vi "XLP80_GUI_PandID.vi"(8 "err in":errorcluster) -> (0 "err out":errorcluster)   [LabVIEW 2021]
uses:
  XLP80_ProjectLibs/XLP80_GUI_V001.llb/XLP80_GUI_TDefClusterPandID_Gen2_FM2.ctl
  XLP80_ProjectLibs/XLP80_GUI_V001.llb/XLP80_GUI_TDefClusterPandID_Gen2_FM1.ctl
  XLP80_ProjectLibs/XLP80_Globals/Globals_Settings_XLP80.vi
  XLP80_General_Libs/WL_Libs_V14.25/WL_Frontpanel_V14.01.llb/WL_Frontpanel_GblStatus.vi
panel:
  out "P&IDs":enum32{"P&ID_GEN2_FM1", "P&ID_GEN2_FM2"}(tab)
  out "P&ID_GEN2_FM1":T1 {"A11_HBV_s_Valve_Act" format="%.1f %"; "A12_SIV_s_Valve_Act" format="%.1f %"; "A13_SOV_s_Valve_Act" format="%.1f %"; "H63_HLD_s_H2_Concentration" format="%.0f ppm"; "H37_GHU_s_Temperature_1" format="%.1f °C"; "H36_GHU_s_Pressure_1" format="%.1f kPa"; "H42_HRB_s_ARB_Spd" format="%.0f rpm"; "H43_HDV_a_Dosing_Valve_Set" format="%.1f %"; "H41_GHU_s_Temperature_2" format="%.1f °C"; "H40_GHU_s_Pressure_2" format="%.1f kPa"; "A23_HSO_s_Humidity" format="%.1f %"; "A17_SO_s_Outlet_Temperature" format="%.1f °C"; "A17_SO_s_Outlet_Pressure" format="%.1f kPa"; "A56_SO_s_Temperature" format="%.1f °C"; "H55_SI_s_Stack_Inlet_Pressure" format="%.1f kPa"; "C08_AMB_s_Humidity_Rel" format="%.1f %"; "C08_AMB_s_Pressure" format="%.1f kPa"; "C08_AMB_s_Temperature" format="%.1f °C"; "H63_HLD_s_H2_Concentration" format="%.0f ppm"; "E71_DC4880_s_Temperature_1_Act" format="%.1f °C"; "E71_DC4880_s_Voltage_In_Actual" format="%.1f V"; "E71_DC4880_s_Voltage_Out_Actual" format="%.1f V"; "E71_DC4880_s_Current_In_Actual" format="%.1f A"; "E71_DC4880_s_Current_Out_Actual" format="%.1f A"; "C54_SI_s_Temperature" format="%.1f °C"; "A15_SI_s_Inlet_Pressure" format="%.1f kPa"; "A16_SI_s_Inlet_Temperature" format="%.1f °C"; "A22_HSI_s_Humidity" format="%.1f %"; "A14_HFM_s_Temperature" format="%.1f °C"; "A14_HFM_s_Pressure" format="%.1f kPa"; "A14_HFM_s_AirMassFlow" format="%.1f g/s"; "A14_HFM_s_Humidity" format="%.1f %"; "A03_ETC_s_Speed_Actual" format="%.0f rpm"; "C04_DI_s_Temperature" format="%.1f °C"; "C02_CP_a_RPM" format="%.1f %"; "C01_RF_a_FanSpeed" format="%.1f %"; "C07_BAT_s_System_Current" format="%.1f A"; "C07_BAT_s_External_Load_Voltage" format="%.1f V"; "C07_BAT_s_Board_Temperature" format="%.1f °C"}
  out "P&ID_GEN2_FM2":T2 {"A11_HBV_s_Valve_Act" format="%.1f %"; "H45_WT_s_WaterLevelStatus" format="%.1f %"; "H63_HLD_s_concH2_FM2" format="%.1f %"; "C24_TRO_s_Temperature_FM23" format="%.1f °C"; "C29_TSO_s_Temperature_FM3" format="%.1f °C"; "H31_OTV_s_Pressure_FM12" format="%.1f kPa"; "H31_OTV_s_Temperature" format="%.1f °C"; "A13_SOV_s_Valve_Act" format="%.1f %"; "H36_GHU_s_Pressure_1_FM12" format="%.1f kPa"; "H42_HRB_s_ARB_Spd" format="%.0f rpm"; "H43_HDV_a_Dosing_Valve_Set" format="%.1f %"; "H41_GHU_s_Temperature_2" format="%.1f °C"; "H40_GHU_s_Pressure_2_FM12" format="%.1f kPa"; "A17_SO_s_Outlet_Temperature" format="%.1f °C"; "A17_SO_s_Outlet_Pressure_FM12" format="%.1f kPa"; "A56_SO_s_Temperature" format="%.1f °C"; "H55_SI_s_Stack_Inlet_Pressure" format="%.1f kPa"; "C08_AMB_s_Humidity_Rel" format="%.1f %"; "C08_AMB_s_Pressure" format="%.1f kPa"; "C08_AMB_s_Temperature" format="%.1f °C"; "H62_HLD_s_H2_Concentration" format="%.0f ppm"; "E71_DC4880_s_Temperature_1_Act" format="%.1f °C"; "E71_DC4880_s_Voltage_In_Actual" format="%.1f V"; "E71_DC4880_s_Voltage_Out_Actual" format="%.1f V"; "E71_DC4880_s_Current_In_Actual" format="%.1f A"; "E71_DC4880_s_Current_Out_Actual" format="%.1f A"; "C54_SI_s_Temperature" format="%.1f °C"; "A15_SI_s_Inlet_Pressure_FM12" format="%.1f kPa"; "A15_SI_s_Inlet_Temperature" format="%.1f °C"; "A22_HSI_s_Humidity_FM12" format="%.1f %"; "A14_HFM_s_Temperature" format="%.1f °C"; "A14_HFM_s_Pressure" format="%.1f kPa"; "A14_HFM_s_AirMassFlow" format="%.1f g/s"; "A14_HFM_s_Humidity" format="%.1f %"; "A03_ETC_s_Speed_Actual" format="%.0f rpm"; "C04_DI_s_Temperature" format="%.1f °C"; "C02_CP_s_ACTUAL_SPEED_FM2" format="%.0f rpm"; "C01_RF_a_FanSpeed" format="%.1f %"; "C07_BAT_s_System_Current" format="%.1f A"; "C07_BAT_s_External_Load_Voltage" format="%.1f V"; "C07_BAT_s_Board_Temperature" format="%.1f °C"}
  in  "but_Close":bool
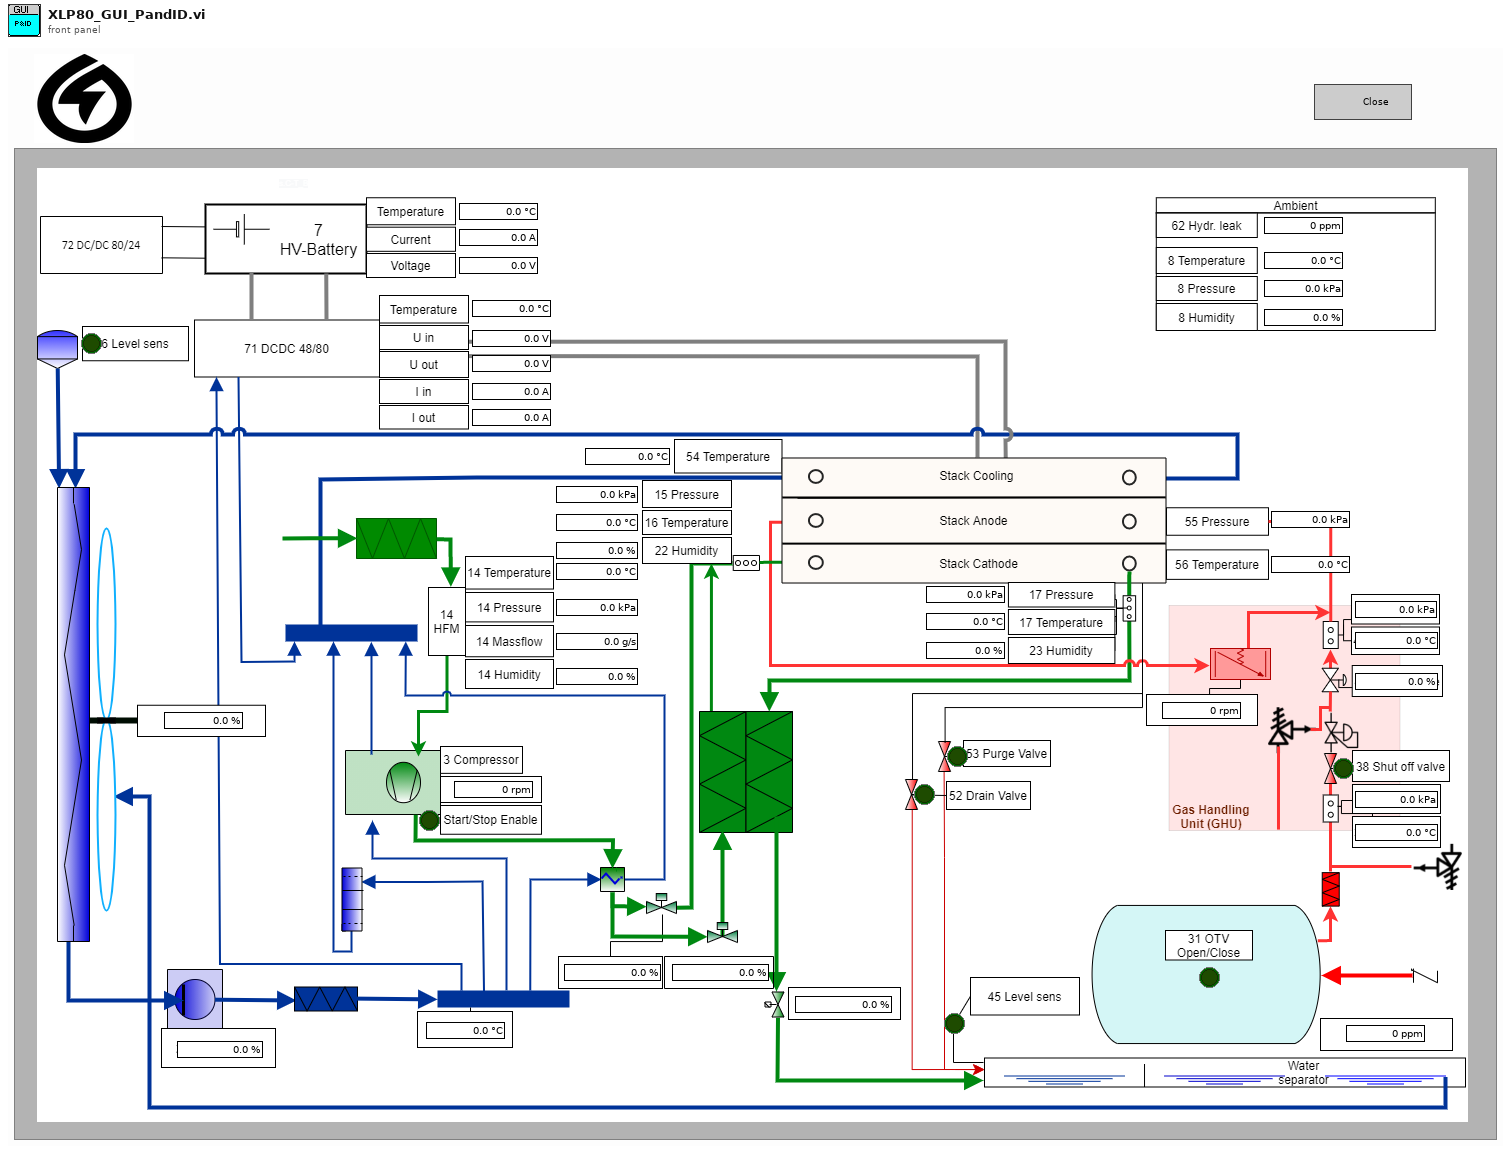
[diagram p1: front panel]
types:
  T1 = typedef "XLP80_GUI_TDefClusterPandID_Gen2_FM1.ctl" = cluster{"C07_BAT_s_Board_Temperature":dbl, "C07_BAT_s_External_Load_Voltage":dbl, "C07_BAT_s_System_Current":dbl, "C06_ET_s_CoolLevelStatus":bool, "C01_RF_a_FanSpeed":dbl, "C02_CP_a_RPM":dbl, "C04_DI_s_Temperature":dbl, "A03_ETC_a_opCmd1_Start_Stop":bool, "A03_ETC_s_Speed_Actual":dbl, "A14_HFM_s_Humidity":dbl, "A14_HFM_s_AirMassFlow":dbl, "A14_HFM_s_Pressure":dbl, "A14_HFM_s_Temperature":dbl, "A22_HSI_s_Humidity":dbl, "A16_SI_s_Inlet_Temperature":dbl, "A15_SI_s_Inlet_Pressure":dbl, "C54_SI_s_Temperature":dbl, "E71_DC4880_s_Current_Out_Actual":dbl, "E71_DC4880_s_Current_In_Actual":dbl, "E71_DC4880_s_Voltage_Out_Actual":dbl, "E71_DC4880_s_Voltage_In_Actual":dbl, "E71_DC4880_s_Temperature_1_Act":dbl, "H63_HLD_s_H2_Concentration":dbl, "C08_AMB_s_Temperature":dbl, "C08_AMB_s_Pressure":dbl, "C08_AMB_s_Humidity_Rel":dbl, "H55_SI_s_Stack_Inlet_Pressure":dbl, "A56_SO_s_Temperature":dbl, "A17_SO_s_Outlet_Pressure":dbl, "A17_SO_s_Outlet_Temperature":dbl, "A23_HSO_s_Humidity":dbl, "H40_GHU_s_Pressure_2":dbl, "H41_GHU_s_Temperature_2":dbl, "H43_HDV_a_Dosing_Valve_Set":dbl, "H42_HRB_s_ARB_Spd":dbl, "H52_DV_a_Drain_Valve_Stack_Set":bool, "H53_PV_a_Purge_Valve_Stack_Set":bool, "H38_HSV_a_Valve_Set":bool, "H36_GHU_s_Pressure_1":dbl, "H37_GHU_s_Temperature_1":dbl, "H31_OTV_a_Valve_Set":bool, "H63_HLD_s_H2_Concentration":dbl, "H45_WT_s_WaterLevelStatus":bool, "A13_SOV_s_Valve_Act":dbl, "A12_SIV_s_Valve_Act":dbl, "A11_HBV_s_Valve_Act":dbl}
  T2 = typedef "XLP80_GUI_TDefClusterPandID_Gen2_FM2.ctl" = cluster{"C07_BAT_s_Board_Temperature":dbl, "C07_BAT_s_External_Load_Voltage":dbl, "C07_BAT_s_System_Current":dbl, "C06_ET_s_CoolLevelStatus":bool, "C01_RF_a_FanSpeed":dbl, "C02_CP_s_ACTUAL_SPEED_FM2":dbl, "C04_DI_s_Temperature":dbl, "A03_ETC_a_opCmd1_Start_Stop":bool, "A03_ETC_s_Speed_Actual":dbl, "A14_HFM_s_Humidity":dbl, "A14_HFM_s_AirMassFlow":dbl, "A14_HFM_s_Pressure":dbl, "A14_HFM_s_Temperature":dbl, "A22_HSI_s_Humidity_FM12":dbl, "A15_SI_s_Inlet_Temperature":dbl, "A15_SI_s_Inlet_Pressure_FM12":dbl, "C54_SI_s_Temperature":dbl, "E71_DC4880_s_Current_Out_Actual":dbl, "E71_DC4880_s_Current_In_Actual":dbl, "E71_DC4880_s_Voltage_Out_Actual":dbl, "E71_DC4880_s_Voltage_In_Actual":dbl, "E71_DC4880_s_Temperature_1_Act":dbl, "H62_HLD_s_H2_Concentration":dbl, "C08_AMB_s_Temperature":dbl, "C08_AMB_s_Pressure":dbl, "C08_AMB_s_Humidity_Rel":dbl, "H55_SI_s_Stack_Inlet_Pressure":dbl, "A56_SO_s_Temperature":dbl, "A17_SO_s_Outlet_Pressure_FM12":dbl, "A17_SO_s_Outlet_Temperature":dbl, "H40_GHU_s_Pressure_2_FM12":dbl, "H41_GHU_s_Temperature_2":dbl, "H43_HDV_a_Dosing_Valve_Set":dbl, "H42_HRB_s_ARB_Spd":dbl, "H52_DV_a_Drain_Valve_Stack_Set":bool, "H53_PV_a_Purge_Valve_Stack_Set":bool, "H38_HSV_a_Valve_Set":bool, "H36_GHU_s_Pressure_1_FM12":dbl, "H31_OTV_a_Valve_Set":bool, "A13_SOV_s_Valve_Act":dbl, "H31_OTV_s_Temperature":dbl, "H31_OTV_s_Pressure_FM12":dbl, "E_76_HVM_a_Relais_Set":bool, "E_75_HVP_a_Relais_Set":bool, "C61_SV_a_FanEnable_FM2":bool, "C29_TSO_s_Temperature_FM3":dbl, "C02_CP_a_ENABLE_FM2":bool, "C24_TRO_s_Temperature_FM23":dbl, "H63_HLD_s_concH2_FM2":dbl, "C27_RIV_a_Valve_Set_FM2":bool, "C28_RBV_a_Valve_Set_FM2":bool, "H45_WT_s_WaterLevelStatus":dbl, "A11_HBV_s_Valve_Act":dbl}
  T3 = enum32{"Invalid", "Standard", "Closed", "Hidden", "Minimized", "Maximized"}
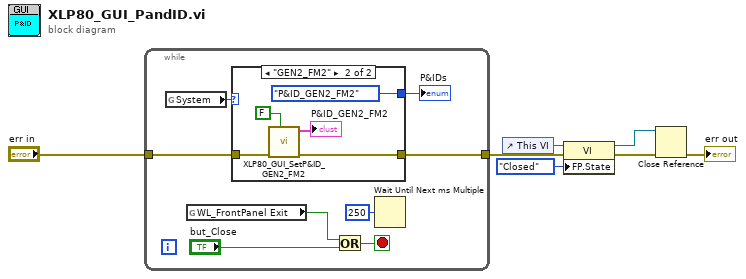
[diagram p0: block diagram]
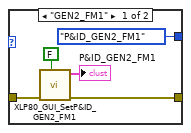
[diagram p2: hidden frame]
diagram:
  n1 = while {
    tunnel: "err in" -> [w11]
    tunnel: [w10] -> w7
    stop <- w14 stop-if-true
    n2 = global read "Globals_Settings_XLP80.vi" "System"() -> (w9:enum16{"GEN2_FM1", "GEN2_FM2"})
    n3 = global read "WL_Frontpanel_GblStatus.vi" "WL_FrontPanel Exit"() -> (w12:bool)
    n4 = case shown="\"GEN2_FM2\"" w9 {
      tunnel: w11 -> [w19 w25]
      tunnel: [w18 w22] -> w10
      tunnel: [enum32{"P&ID_GEN2_FM1", "P&ID_GEN2_FM2"}."P&ID_GEN2_FM1" ("P&IDs") enum32{"P&ID_GEN2_FM1", "P&ID_GEN2_FM2"}."P&ID_GEN2_FM2" ("P&IDs")] -> w8
      frame "GEN2_FM1" {
        n5 = call "XLP80_GUI_SetP&ID_GEN2_FM1.vi"("SetRef"=FALSE, "err in"=w19) -> ("err out"=w18:errorcluster, "P&ID_GEN2_FM1"=→"P&ID_GEN2_FM1":T1)  [unwired: 8 in]
      }
      frame "GEN2_FM2" {
        n6 = call "XLP80_GUI_SetP&ID_GEN2_FM2.vi"("SetRef"=FALSE, "err in"=w25) -> ("err out"=w22:errorcluster, "P&ID_GEN2_FM2"=→"P&ID_GEN2_FM2":T2)  [unwired: 8 in]
      }
    }
    "P&IDs" <- w8
    n7 = Or(x=w12, y="but_Close") -> (x .or. y?=w14:bool)
    n8 = Wait Until Next ms Multiple(millisecond multiple=u32 250) -> ()  [unwired: 1 out]
  }
  n9 = control-ref of="This VI"() -> (w5:refnum<vi>)
  n10 = property class="VI"(reference=w5, error in=w7, "FP.State"=T3."Closed" ("Front Panel Window:State")) -> (reference out=w2:refnum<vi>, error out=w6:errorcluster)
  n11 = Close Reference(reference=w2, error in (no error)=w6) -> (error out=→"err out":errorcluster)
